vi "Test Asserts.vi"(8 "error in (no error)":errorcluster) -> (0 "error out":errorcluster)   [LabVIEW 2009]
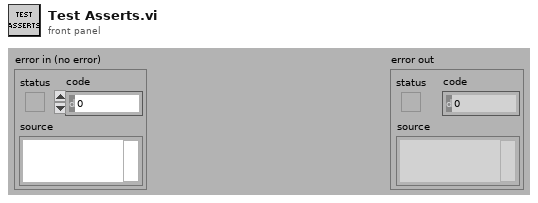
[diagram p1: front panel]
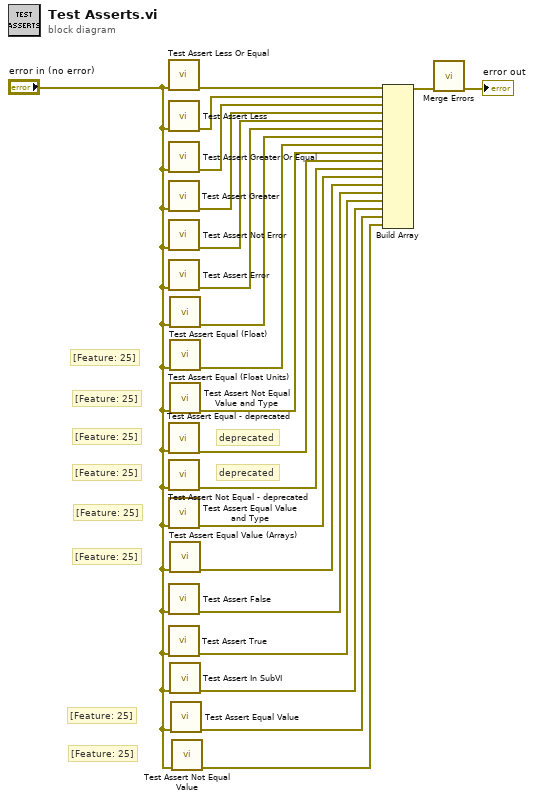
[diagram p0: block diagram]
diagram:
  # "[Feature: 25]"
  # "[Feature: 25]"
  # "[Feature: 25]"
  # "[Feature: 25]"
  # "[Feature: 25]"
  # "[Feature: 25]"
  # "[Feature: 25]"
  # "[Feature: 25]"
  # "deprecated"
  # "deprecated"
  n1 = call "Test Assert Less Or Equal.vi"("error in (no error)"="error in (no error)") -> ("error out"=w21:errorcluster)  [unwired: 10 in]
  n2 = call "Test Assert Less.vi"("error in (no error)"="error in (no error)") -> ("error out"=w20:errorcluster)  [unwired: 10 in]
  n3 = call "Test Assert Greater Or Equal.vi"("error in (no error)"="error in (no error)") -> ("error out"=w19:errorcluster)  [unwired: 10 in]
  n4 = call "Test Assert Greater.vi"("error in (no error)"="error in (no error)") -> ("error out"=w18:errorcluster)  [unwired: 10 in]
  n5 = call "Test Assert Not Error.vi"("error in (no error)"="error in (no error)") -> ("error out"=w17:errorcluster)  [unwired: 10 in]
  n6 = call "Test Assert Error.vi"("error in (no error)"="error in (no error)") -> ("error out"=w16:errorcluster)  [unwired: 10 in]
  n7 = call "Test Assert Equal - deprecated.vi"("error in (no error)"="error in (no error)") -> ("error out"=w6:errorcluster)  [unwired: 10 in]
  n8 = call "Test Assert Not Equal - deprecated.vi"("error in (no error)"="error in (no error)") -> ("error out"=w15:errorcluster)  [unwired: 10 in]
  n9 = call "Test Assert Equal Value and Type.vi"("error in (no error)"="error in (no error)") -> ("error out"=w14:errorcluster)  [unwired: 10 in]
  n10 = call "Test Assert False.vi"("error in (no error)"="error in (no error)") -> ("error out"=w13:errorcluster)  [unwired: 10 in]
  n11 = call "Test Assert True.vi"("error in (no error)"="error in (no error)") -> ("error out"=w12:errorcluster)  [unwired: 10 in]
  n12 = call "Test Assert Equal (Float).vi"("error in (no error)"="error in (no error)") -> ("error out"=w5:errorcluster)  [unwired: 10 in]
  n13 = call "Test Assert Equal (Float Units).vi"("error in (no error)"="error in (no error)") -> ("error out"=w1:errorcluster)  [unwired: 10 in]
  n14 = call "Test Assert Not Equal Value and Type.vi"("error in (no error)"="error in (no error)") -> ("error out"=w4:errorcluster)  [unwired: 10 in]
  n15 = call "Test Assert Equal Value (Arrays).vi"("error in (no error)"="error in (no error)") -> ("error out"=w3:errorcluster)  [unwired: 10 in]
  n16 = call "Test Assert In SubVI.vi"("error in (no error)"="error in (no error)") -> ("error out"=w9:errorcluster)  [unwired: 10 in]
  n17 = call "Test Assert Equal Value.vi"("error in (no error)"="error in (no error)") -> ("error out"=w8:errorcluster)  [unwired: 10 in]
  n18 = call "Test Assert Not Equal Value.vi"("error in (no error)"="error in (no error)") -> ("error out"=w7:errorcluster)  [unwired: 10 in]
  n19 = Build Array(w21, w20, w19, w18, w17, w16, w5, w1, w4, w6, w15, w14, w3, w13, w12, w9, w8, w7) -> (w11:errorcluster[])
  n20 = call <vilib>:"Merge Errors.vi"("error array in"=w11) -> ("error out"=→"error out":errorcluster)  [unwired: 6 in]
